vi "set_config_cluster.vi"(8 "error in (no error)":errorcluster, 10 "config cluster variant":variant, 11 "DisplayDL090216 in":refnum<class "DisplayDL090216.lvclass">) -> (0 "error out":errorcluster, 3 "DisplayDL090216 out":refnum<class "DisplayDL090216.lvclass">)   [LabVIEW 2010, in "DisplayDL090216.lvclass"]
uses:
  DisplayDL090216.lvclass
  DisplayDL090216.lvclass/DisplayDL090216.ctl
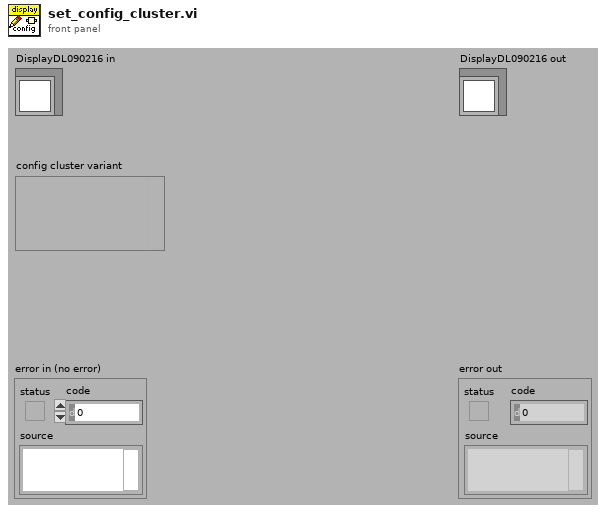
[diagram p1: front panel]
types:
  T1 = typedef "DisplayDL090216.lvclass/config_data_cluster.ctl" = cluster{"image processors":T2[], "range/offset processor configuration":string, "number of channels":i32, "autoscale cluster":cluster{"autoscale histogram":bool, "channel_1_min":dbl, "channel_1_max":dbl, "channel_2_min":dbl, "channel_2_max":dbl, "channel_3_min":dbl, "channel_3_max":dbl}}
  T2 = typedef "plugin_specification.ctl" = cluster{"class path":string, "configuration":string, "label":string, "settings name":string}
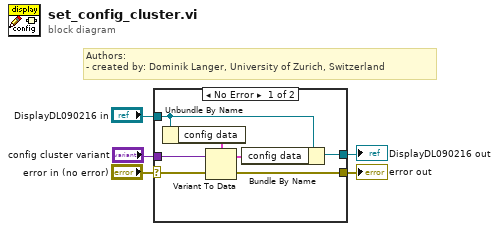
[diagram p0: block diagram]
diagram:
  # "Authors: \n- created by: Dominik Langer, University of Zurich, Switzerland"
  n1 = case shown="No Error" "error in (no error)" {
    selector: "error in (no error)" -> [w10 w13]
    tunnel: "DisplayDL090216 in" -> [w8 w14]
    tunnel: [w7 w13] -> w5
    tunnel: [w6 w14] -> w4
    tunnel: "config cluster variant" -> [w9 _]
    frame No Error {
      n2 = Unbundle By Name(w8) -> ("config data"=w12:T1)
      n3 = Variant To Data(error in=w10, Variant=w9, type=w12) -> (error out=w7:errorcluster, data=w11:T1)
      n4 = Bundle By Name(cluster=w8, "config data"=w11) -> (w6:refnum<class "DisplayDL090216.lvclass">)
    }
    frame Error {
    }
  }
  "error out" <- w5
  "DisplayDL090216 out" <- w4
